vi "Send Panel Refercence.vi"(0 "Microscope in":refnum<class "Microscope.lvclass">, 5 "Sub Panel":string, 9 "VI Refnum":refnum<vi>, 11 "error in (no error)":errorcluster) -> (4 "Microscope out":refnum<class "Microscope.lvclass">, 15 "error out":errorcluster)   [LabVIEW 2020, in "Microscope.lvlib" / "Microscope.lvclass"]
uses:
  Microscope.lvclass
  Microscope.lvclass/Microscope.ctl
  Microscope Controller Messages/Insert Panel To Controller Msg/Insert Panel To Controller Msg.lvclass/Insert Panel To Controller Msg.ctl
  <vilib>/ActorFramework/Message Enqueuer/Message Enqueuer.lvclass/Message Enqueuer.ctl
  <vilib>/ActorFramework/Message Enqueuer/Enqueue.vi
  Microscope Controller Messages/Insert Panel To Controller Msg/Insert Panel To Controller Msg.lvclass
  C:/Program Files/National Instruments/LabVIEW 2020/vi.lib/ActorFramework/Message/Message.lvclass
  <vilib>/ActorFramework/Message Priority Queue/Priority Enqueue.vi
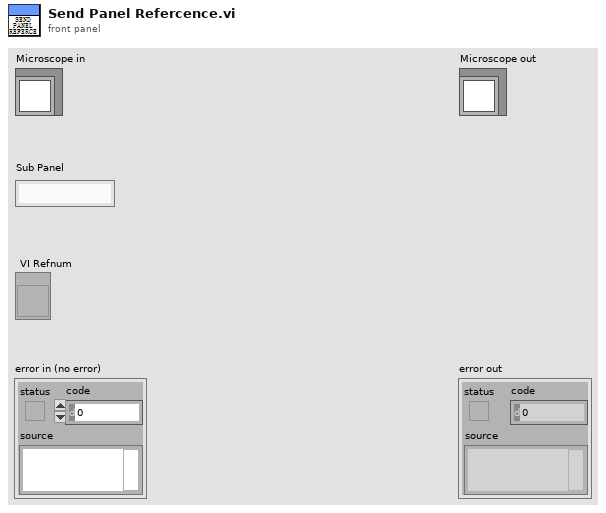
[diagram p1: front panel]
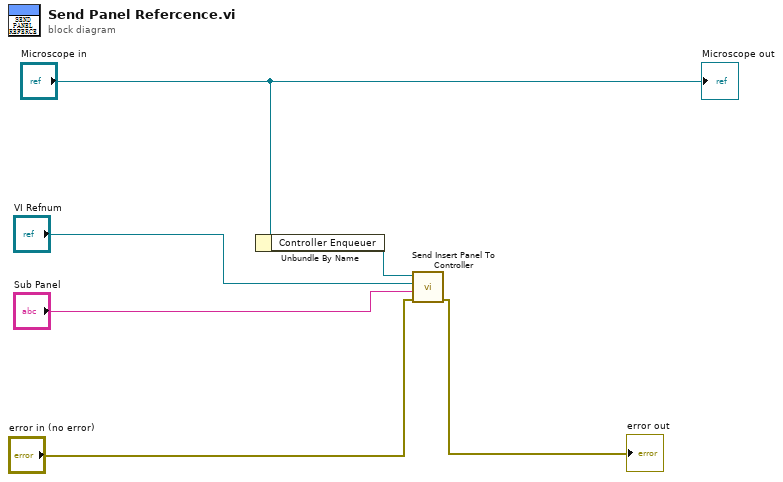
[diagram p0: block diagram]
diagram:
  n1 = Unbundle By Name("Microscope in") -> ("Controller Enqueuer"=w6:refnum<class "Message Enqueuer.lvclass">)
  n2 = call "Send Insert Panel To Controller.vi"("error in (no error)"="error in (no error)", "Sub Panel"="Sub Panel", "VI Refnum"="VI Refnum", "Message Enqueuer"=w6) -> ("error out"=→"error out":errorcluster)  [unwired: 6 in, 1 out]
  "Microscope out" <- "Microscope in"
